vi "1 Tick Pulse.vi"(4 "Input":bool) -> (1 "Output":bool)   [LabVIEW 2018]
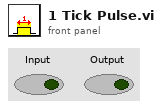
[diagram p1: front panel]
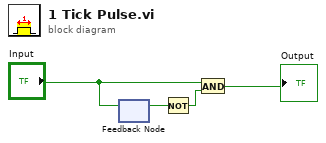
[diagram p0: block diagram]
diagram:
  n1 = feedback-in #1("Input") -> ()
  n2 = feedback #1() -> (w2:bool)  [unwired: 1 in]
  n3 = Not(x=w2) -> (.not. x?=w4:bool)
  n4 = And(x="Input", y=w4) -> (x .and. y?=→"Output":bool)
